vi "Rec Move To Record N (R).vi"(8 "error in (no error)":errorcluster, 10 "n (0)":i32, 11 "recordset reference":T1) -> (0 "error out":errorcluster, 3 "recordset reference out":T1)   [LabVIEW 2013, in "NI_Database_API_64.lvlib"]
doc: "Moves the cursor to point to record <B>n</B> in the recordset. To move the cursor to the last record, set <B>n</B> to -1. You cannot use this VI with a forward-only cursor. Wire data to the reference input to determine the polymorphic instance to use or manually select the instance."
uses:
  NI_Database_API_64.lvlib
  Rec ObjectReference.ctl
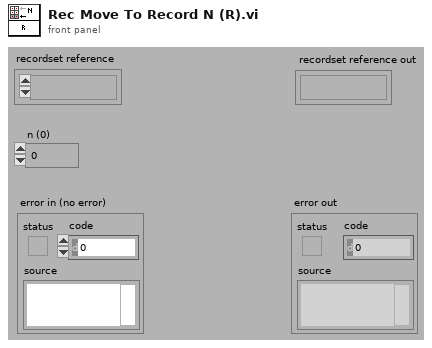
[diagram p1: front panel]
types:
  T1 = typedef "NI_Database_API_64.lvlib/Rec ObjectReference.ctl" = refnum<k1>
  T2 = typedef "NI_Database_API_64.lvlib/Rec DataMembers.ctl" = cluster{"ADODB._Recordset":refnum<k7>, "Connection":T3}
  T3 = typedef "NI_Database_API_64.lvlib/Conn ObjectReference.ctl" = refnum<k1>
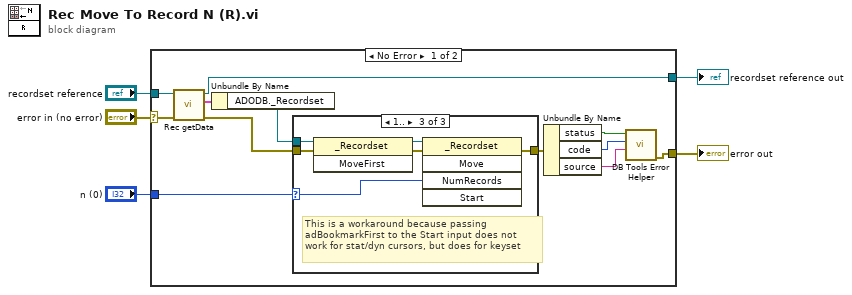
[diagram p0: block diagram]
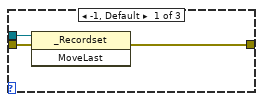
[diagram p2: hidden frame]
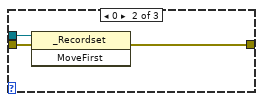
[diagram p3: hidden frame]
diagram:
  n1 = case shown="No Error" "error in (no error)" {
    selector: "error in (no error)" -> [w6 w31]
    tunnel: "recordset reference" -> [w17 w30]
    tunnel: "n (0)" -> [w16 _]
    tunnel: [w12 w30] -> w3
    tunnel: [w7 w31] -> w2
    frame No Error {
      n2 = call "Rec getData.vi"("error in (no error)"=w6, "recordset reference"=w17) -> ("error out"=w14:errorcluster, "data"=w15:T2, "recordset reference out"=w12:T1)  [unwired: 3 out]
      n3 = Unbundle By Name(w15) -> ("ADODB._Recordset"=w13:refnum<k7>)
      n4 = case shown="1.." w16 {
        selector: w16 -> [_ _ w24]
        tunnel: [w20 w23 w27] -> w8
        tunnel: w14 -> [w19 w22 w29]
        tunnel: w13 -> [w18 w21 w28]
        frame -1, Default {
          n5 = invoke class="_Recordset" method="MoveLast"(reference=w18, error in=w19) -> (error out=w20:errorcluster)  [unwired: 1 in, 2 out]
        }
        frame 0 {
          n6 = invoke class="_Recordset" method="MoveFirst"(reference=w21, error in=w22) -> (error out=w23:errorcluster)  [unwired: 1 in, 2 out]
        }
        frame 1.. {
          # "This is a workaround because passing\nadBookmarkFirst to the Start input does not\nwork for stat/dyn cursors, but does for keyset"
          n7 = invoke class="_Recordset" method="MoveFirst"(reference=w28, error in=w29) -> (reference out=w26:refnum<k7>, error out=w25:errorcluster)  [unwired: 1 in, 1 out]
          n8 = invoke class="_Recordset" method="Move"(reference=w26, error in=w25, "NumRecords"=w24) -> (error out=w27:errorcluster)  [unwired: 2 in, 4 out]
        }
      }
      n9 = Unbundle By Name(w8) -> ("status"=w10:bool, "code"=w9:i32, "source"=w11:string)
      n10 = call "DB Tools Error Helper.vi"("source"=w11, "code"=w9, "status"=w10) -> ("error out"=w7:errorcluster)  [unwired: 1 in, 7 out]
    }
    frame Error {
    }
  }
  "recordset reference out" <- w3
  "error out" <- w2
